vi "GetClusterElementIndices.vi"(5 "Element Name":string[](array[string]), 6 "error in":errorcluster, 9 "Cluster":variant) -> (0 "error out":errorcluster, 4 "indices":i32[](array[numeric]))   [LabVIEW 2014]
uses:
  <vilib>/Utility/VariantDataType/VariantType.lvlib
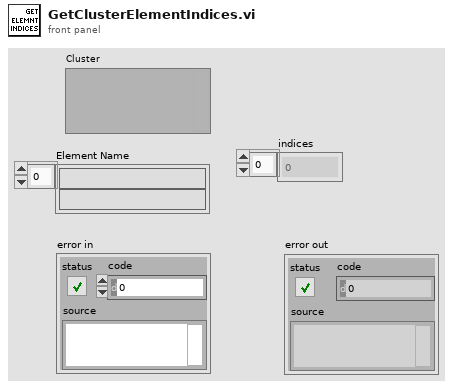
[diagram p1: front panel]
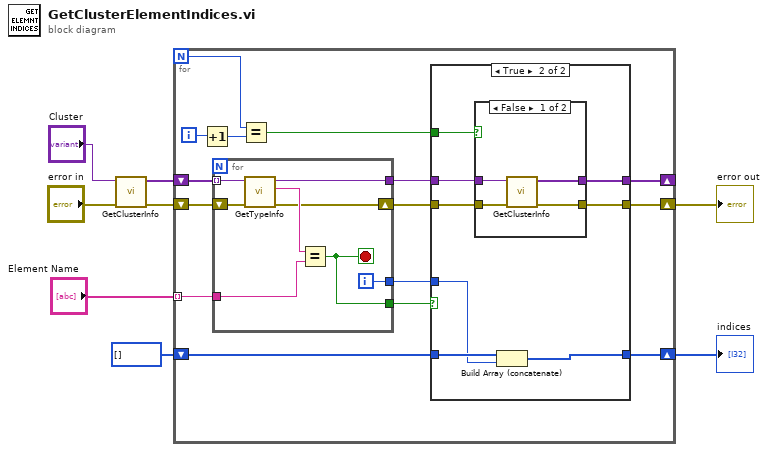
[diagram p0: block diagram]
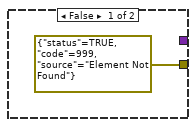
[diagram p2: hidden frame]
diagram:
  n1 = call <vilib>:"GetClusterInfo.vi"("error in (no error)"="error in", "Variant"="Cluster") -> ("error out"=w1:errorcluster, "Cluster Elements"=w2:variant[])  [unwired: 8 in]
  n2 = for {
    N -> [w19]
    tunnel: "Element Name" -> [w22] mode=indexing
    shift-right: [w16] -> _
    shift-left: w2 -> [w23]
    shift-right: [w13] -> w5
    shift-left: w1 -> [w15]
    shift-right: [w9] -> w6
    shift-left: i32[] [] -> [w10]
    i -> [w21]
    n3 = Increment(x=w21) -> (x+1=w20:i32)
    n4 = for {
      tunnel: w23 -> [w38] mode=indexing
      tunnel: w22 -> [w44]
      tunnel: [w38] -> w17
      tunnel: [w42] -> w11
      tunnel: [w41] -> w12
      shift-right: [w40] -> w14
      shift-left: w15 -> [w39]
      i -> [w42]
      stop <- w41 stop-if-true
      n5 = call <vilib>:"GetTypeInfo.vi"("error in (no error)"=w39, "Variant"=w38) -> ("error out"=w40:errorcluster, "Name"=w43:string)  [unwired: 5 in, 3 out]
      n6 = Equal?(x=w43, y=w44) -> (x = y?=w41:bool)
    }
    n7 = Equal?(x=w19, y=w20) -> (x = y?=w18:bool)
    n8 = case shown="True" w12 {
      tunnel: w18 -> [_ w32]
      tunnel: w17 -> [_ w31]
      tunnel: [_ w30] -> w16
      tunnel: w14 -> [_ w29]
      tunnel: [errorcluster {"status"=TRUE, "code"=999, "source"="Element Not Found"} ("error out") w28] -> w13
      tunnel: w11 -> [_ w25]
      tunnel: w10 -> [_ w27]
      tunnel: [_ w26] -> w9
      frame False {
      }
      frame True {
        n9 = case shown="False" w32 {
          tunnel: w31 -> [w35 _]
          tunnel: [w34 _] -> w30
          tunnel: w29 -> [w36 w37]
          tunnel: [w33 w37] -> w28
          frame False {
            n10 = call <vilib>:"GetClusterInfo.vi"("error in (no error)"=w36, "Variant"=w35) -> ("error out"=w33:errorcluster, "Cluster Elements"=w34:variant[])  [unwired: 8 in]
          }
          frame True {
          }
        }
        n11 = Build Array (concatenate)(w27, w25) -> (w26:i32[])
      }
    }
  }
  "indices" <- w6
  "error out" <- w5
